vi "DSC TSV to PGSQL Choose Column Dialog.vi"(8 "error in":errorcluster, 9 "Message":string, 10 "DSC":string, 11 "Item Names":string[](array[string])) -> (0 "error out":errorcluster, 3 "Selection":string)   [LabVIEW 2019]
uses:
  <vilib>/ErrorRing/Error Ring.xnode
panel:
  in  "CANCEL":bool
  in  "Listbox":i32(listbox)
  in  "OK":bool
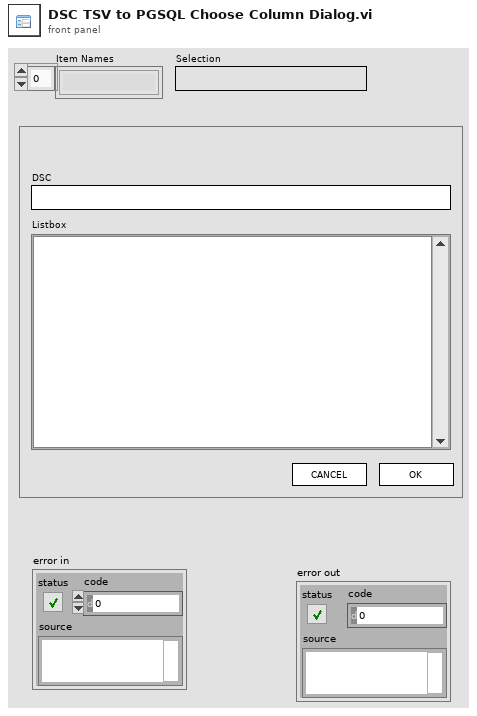
[diagram p1: front panel]
types:
  T1 = enum32{"Invalid", "Standard", "Closed", "Hidden", "Minimized", "Maximized"}
  T2 = enum32{"invalid app kind", "Development System", "Run Time System", "Student Edition", "Embedded LabVIEW", "Evaluation", "Custom"}
  T3 = cluster{"Core":cluster{"Current VI Reference":refnum<vi>, "Close Panel on Exit?":bool}, "Cancel?":bool, "Your string data":string}
  T4 = cluster{"Current VI Reference":refnum<vi>, "Close Panel on Exit?":bool}
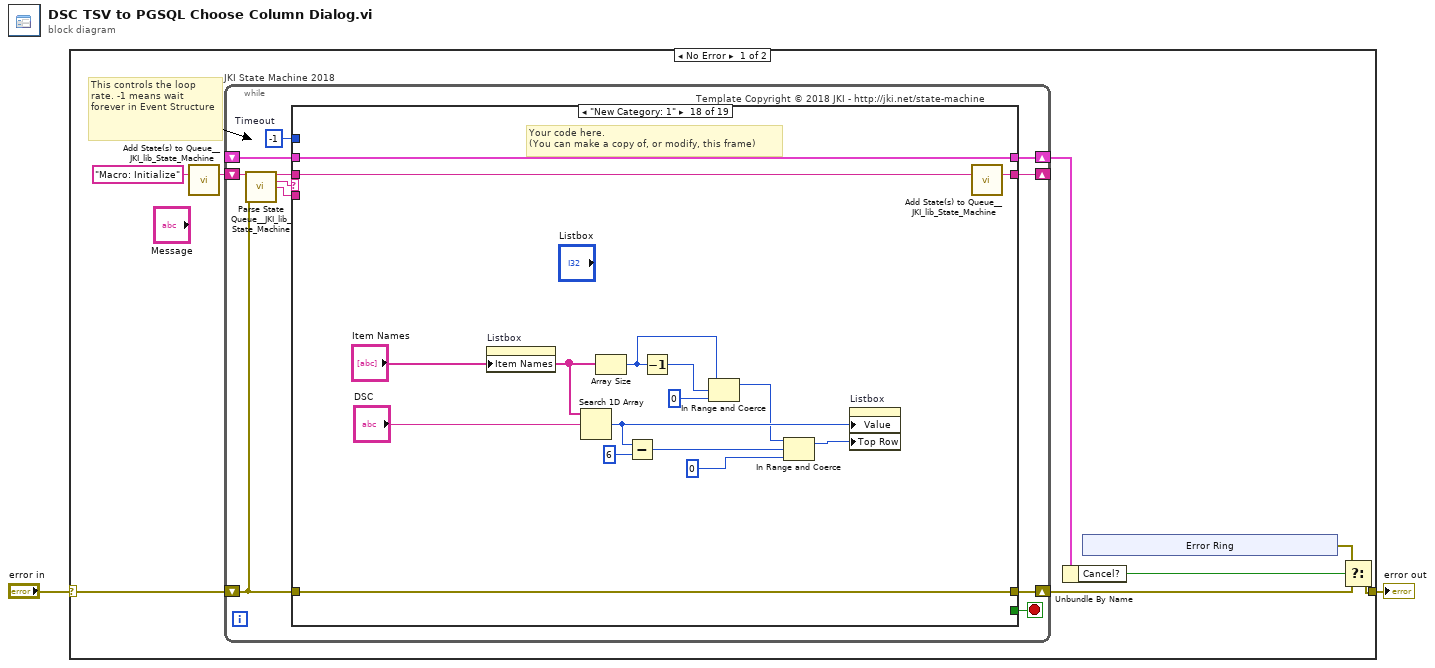
[diagram p0: block diagram]
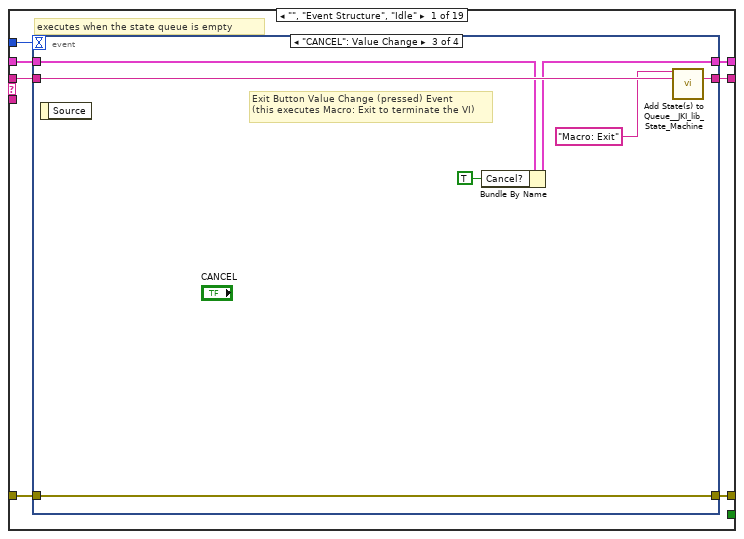
[diagram p2: hidden frame]
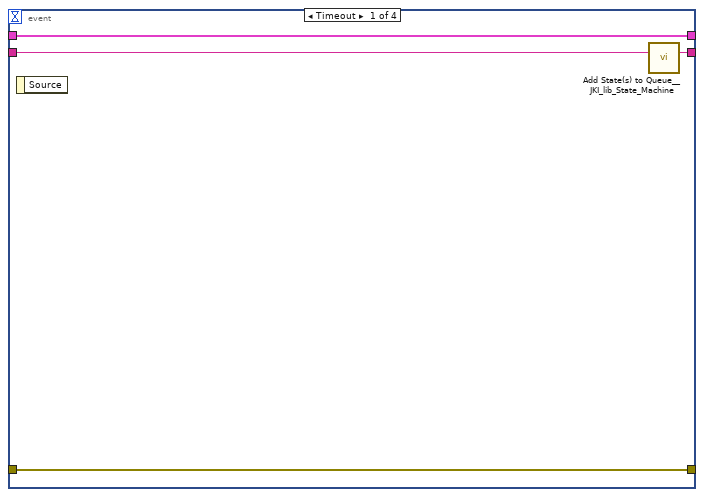
[diagram p3: hidden frame]
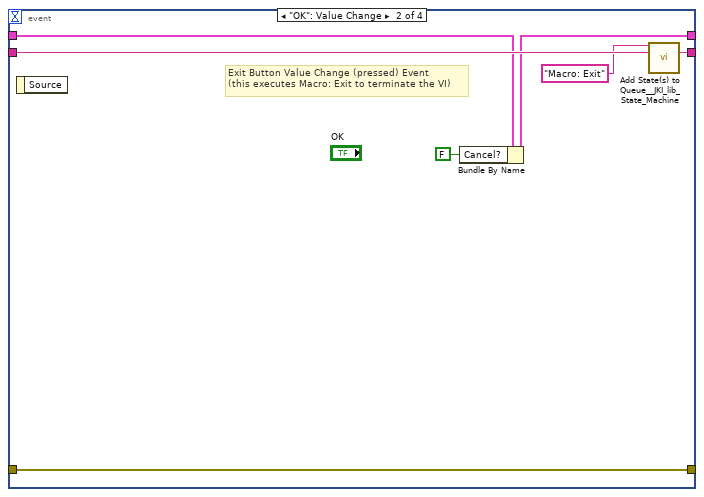
[diagram p4: hidden frame]
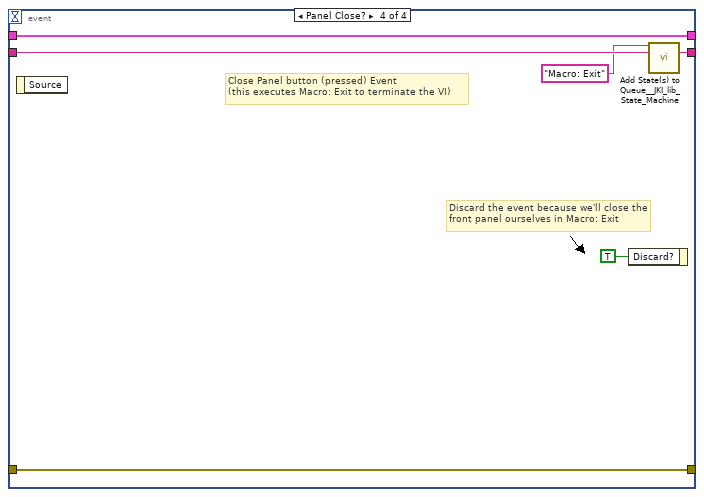
[diagram p5: hidden frame]
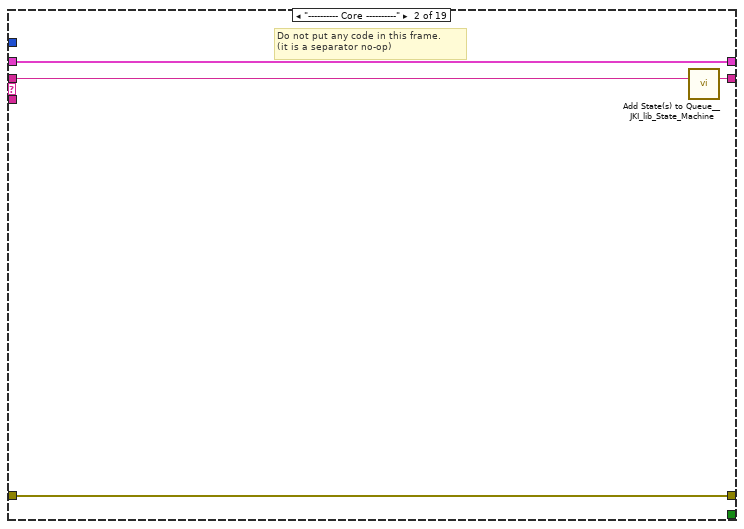
[diagram p6: hidden frame]
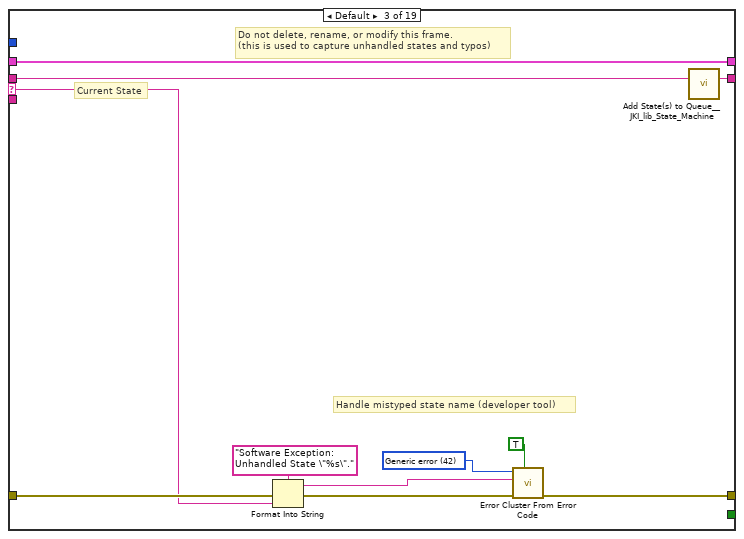
[diagram p7: hidden frame]
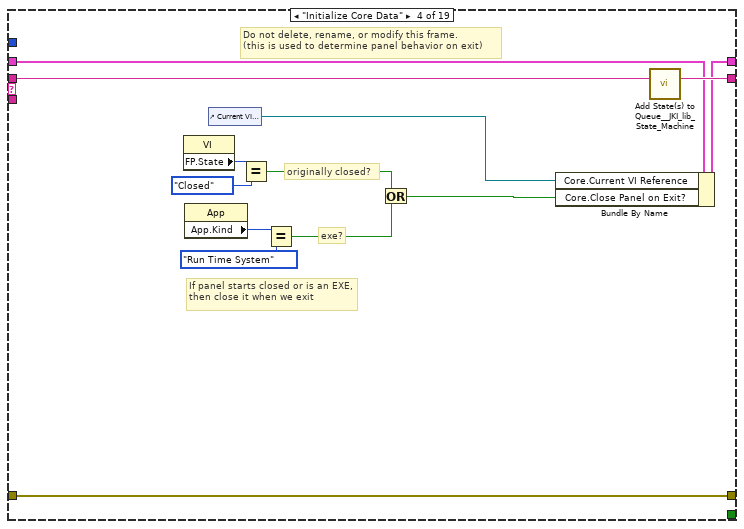
[diagram p8: hidden frame]
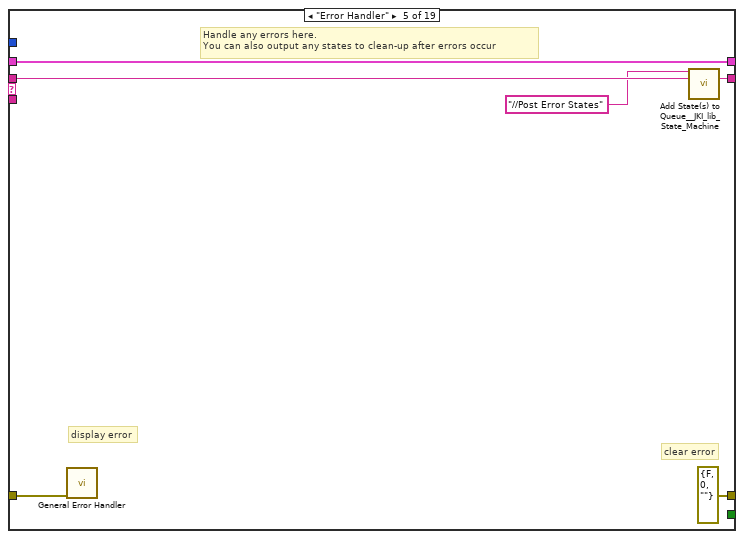
[diagram p9: hidden frame]
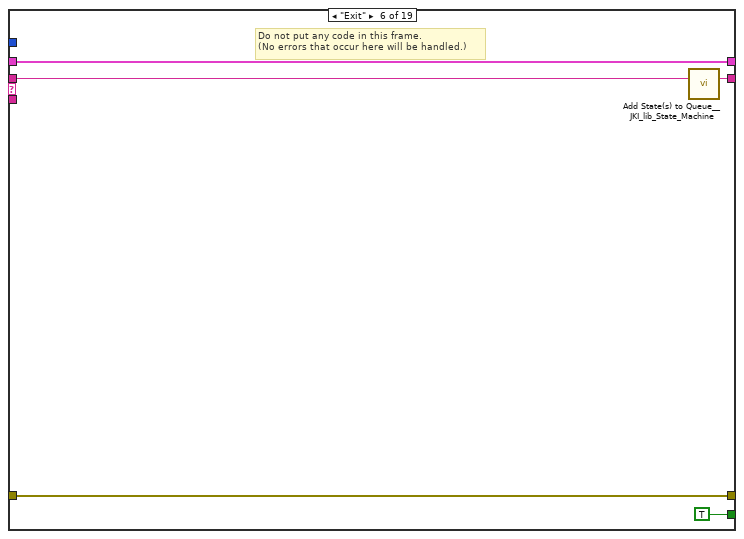
[diagram p10: hidden frame]
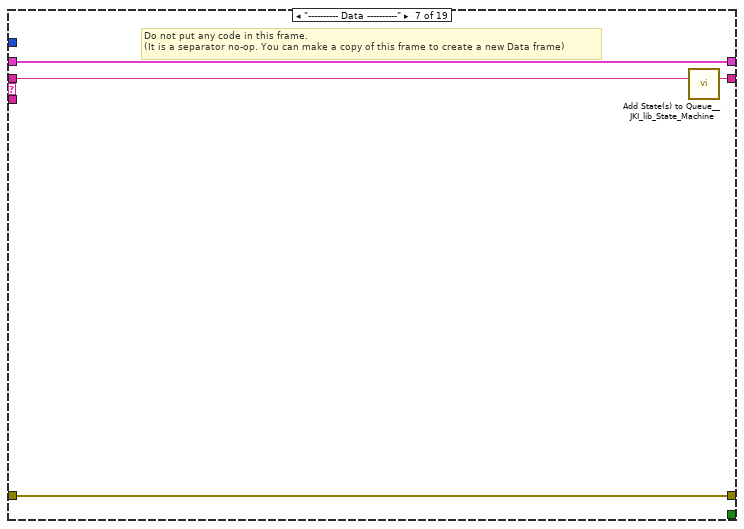
[diagram p11: hidden frame]
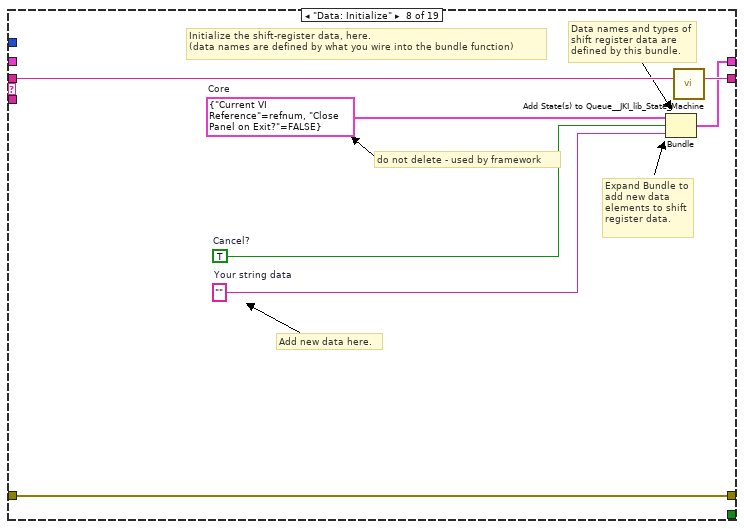
[diagram p12: hidden frame]
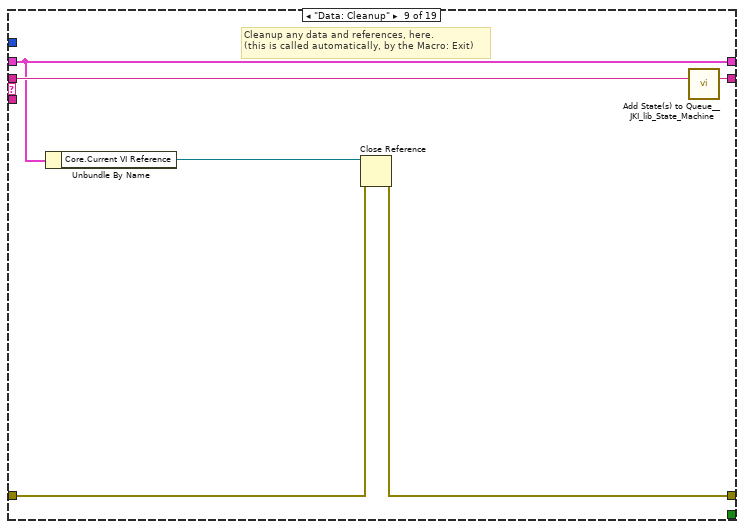
[diagram p13: hidden frame]
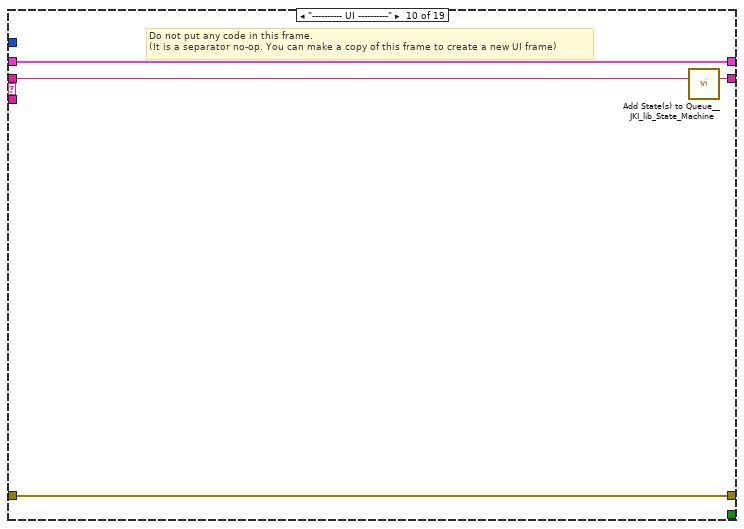
[diagram p14: hidden frame]
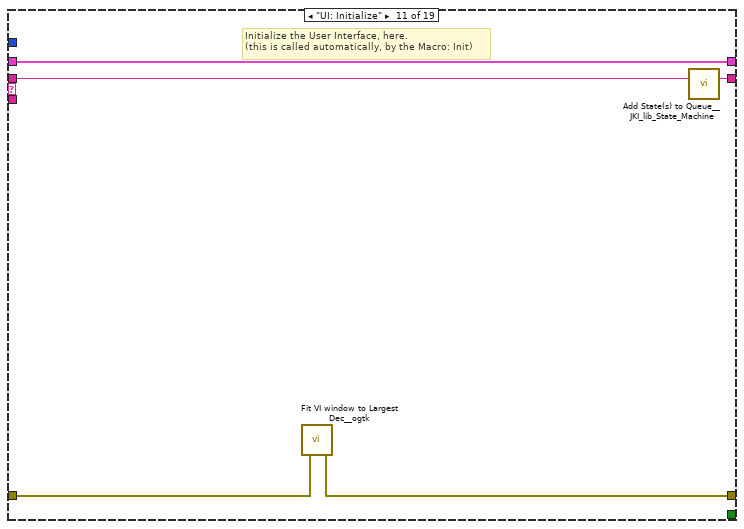
[diagram p15: hidden frame]
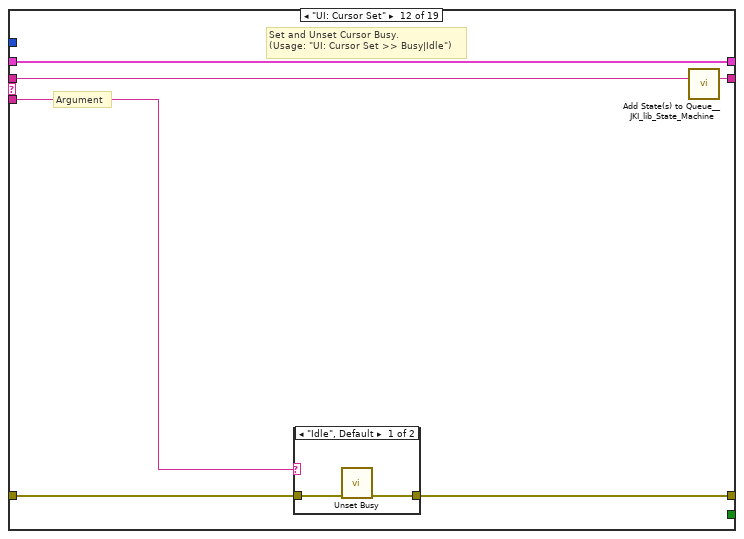
[diagram p16: hidden frame]
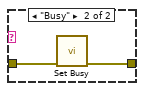
[diagram p17: hidden frame]
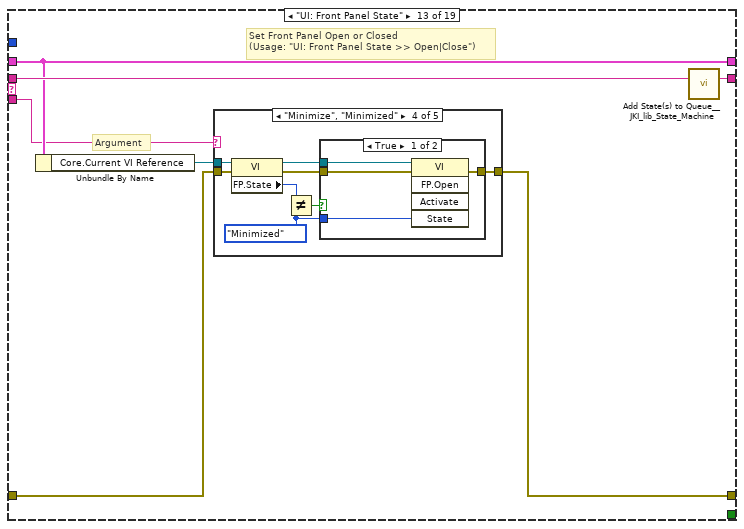
[diagram p18: hidden frame]
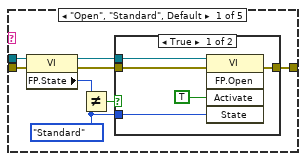
[diagram p19: hidden frame]
diagram:
  n1 = case shown="No Error" "error in" {
    selector: "error in" -> [w3 w250]
    tunnel: [w5 w250] -> w2
    frame No Error {
      # "This controls the loop rate. -1 means wait forever in Event Structure"
      n2 = call <vilib>:"Add State(s) to Queue__JKI_lib_State_Machine.vi"("State(s) in (\"\")"="Macro: Initialize") -> ("States Out"=w10:string)  [unwired: 14 in]
      n3 = while "JKI State Machine 2018" {
        shift-right: [w18] -> w8
        shift-left: _ -> [w17]
        shift-right: [w21] -> w6
        shift-left: w3 -> [w15]
        shift-right: [w20] -> _
        shift-left: w10 -> [w22]
        stop <- w19 stop-if-true
        w16 = -1  # Timeout
        # "Template Copyright © 2018 JKI - http://jki.net/state-machine"
        n4 = call <vilib>:"Parse State Queue__JKI_lib_State_Machine.vi"("State Queue"=w22, "Error In (no error)"=w15) -> ("Remaining States"=w24:string, "Current State"=w25:string, "Arguments"=w23:string)  [unwired: 11 in]
        n5 = case shown="\"New Category: 1\"" w25 {
          selector: w25 -> [_ _ w61 _ _ _ _ _ _ _ _ _ _ _ _ _ _ _ _]
          tunnel: w24 -> [w32 w60 w65 w84 w90 w95 w99 w106 w112 w116 w121 w127 w138 w207 w212 w223 w227 w242 w249]
          tunnel: w23 -> [_ _ _ _ _ _ _ _ _ _ _ w122 w132 _ _ _ _ _ _]
          tunnel: w17 -> [w30 w57 w63 w77 w88 w93 w96 _ w107 w113 w119 w125 w134 w204 w209 w220 w224 w239 w246]
          tunnel: [w29 w58 w67 w81 errorcluster {"status"=FALSE, "code"=0, "source"=""} ("error in") w92 w97 w103 w108 w114 w118 w123 w135 w205 w210 w221 w225 w240 w247] -> w21
          tunnel: w15 -> [w28 w58 w66 w81 w85 w92 w97 w103 w109 w114 w117 w124 w136 w205 w210 w221 w225 w240 w247]
          tunnel: [w31 w59 w64 w83 w89 w94 w98 w105 w111 w115 w120 w126 w137 w206 w211 w222 w226 w241 w248] -> w20
          tunnel: [_ _ _ _ _ TRUE _ _ _ _ _ _ _ _ _ _ _ _ _] -> w19
          tunnel: [w27 w57 w63 w82 w88 w93 w96 w104 w107 w113 w119 w125 w134 w204 w209 w220 w224 w239 w246] -> w18
          tunnel: w16 -> [w26 _ _ _ _ _ _ _ _ _ _ _ _ _ _ _ _ _ _]
          frame "", "Event Structure", "Idle" {
            # "executes when the state queue is empty"
            n6 = event shown="[2] \"CANCEL\": Value Change" {
              selector: _ -> [_ _ _ _]
              dyn-events: _ -> [_ _ _ _]
              timeout: w26 -> [_ _ _ _]
              tunnel: w32 -> [w36 w43 w50 w56]
              tunnel: [w35 w42 w49 w55] -> w31
              tunnel: w30 -> [w33 w37 w44 w53]
              tunnel: [w34 w41 w48 w54] -> w29
              tunnel: w28 -> [w34 w41 w48 w54]
              tunnel: [w33 w38 w45 w53] -> w27
              event Timeout {
                n7 = event-data() -> ()  [unwired: 1 in, 1 out]
                n8 = call <vilib>:"Add State(s) to Queue__JKI_lib_State_Machine.vi"("State(s) in (\"\")"=w36) -> ("States Out"=w35:string)  [unwired: 14 in]
              }
              event "OK": Value Change {
                # "Exit Button Value Change (pressed) Event\n(this executes Macro: Exit to terminate the VI)"
                n9 = event-data() -> ()  [unwired: 1 in, 1 out]
                n10 = Bundle By Name(cluster=w37, "Cancel?"=FALSE) -> (w38:T3)
                n11 = call <vilib>:"Add State(s) to Queue__JKI_lib_State_Machine.vi"("State(s) in Front (\"\")"="Macro: Exit", "State(s) in (\"\")"=w43) -> ("States Out"=w42:string)  [unwired: 13 in]
              }
              event "CANCEL": Value Change {
                # "Exit Button Value Change (pressed) Event\n(this executes Macro: Exit to terminate the VI)"
                n12 = event-data() -> ()  [unwired: 1 in, 1 out]
                n13 = Bundle By Name(cluster=w44, "Cancel?"=TRUE) -> (w45:T3)
                n14 = call <vilib>:"Add State(s) to Queue__JKI_lib_State_Machine.vi"("State(s) in Front (\"\")"="Macro: Exit", "State(s) in (\"\")"=w50) -> ("States Out"=w49:string)  [unwired: 13 in]
              }
              event Panel Close? {
                # "Discard the event because we'll close the front panel ourselves in Macro: Exit"
                # "Close Panel button (pressed) Event\n(this executes Macro: Exit to terminate the VI)"
                n15 = event-data() -> ()  [unwired: 1 in, 1 out]
                n16 = event-data("Discard?"=TRUE) -> ()  [unwired: 1 in, 1 out]
                n17 = call <vilib>:"Add State(s) to Queue__JKI_lib_State_Machine.vi"("State(s) in Front (\"\")"="Macro: Exit", "State(s) in (\"\")"=w56) -> ("States Out"=w55:string)  [unwired: 13 in]
              }
            }
          }
          frame "---------- Core ----------" {
            # "Do not put any code in this frame.\n(it is a separator no-op)"
            n18 = call <vilib>:"Add State(s) to Queue__JKI_lib_State_Machine.vi"("State(s) in (\"\")"=w60) -> ("States Out"=w59:string)  [unwired: 14 in]
          }
          frame Default {
            w70 = 42 items=["No error", "Argument error", "Memory is full", "Out of zone", "End of file", "File already open", "Generic file I/O error", "File not found", "File permission error", "Disk is full", "Duplicate path", "Too many files open", "System feature not enabled", "Resource file not found", "Cannot add resource", "Resource not found", "Image not found", "Image memory error", "Pen does not exist", "Config type invalid", "Config token not found", "Config parse error", "Config memory error", "Bad external code format", "Bad external code offset", "External code not present", "Null window", "Destroy window error", "Null menu", "Print aborted", "Bad print record", "Print driver error", "Windows error during printing", "Memory error during printing", "Print dialog error", "Generic print error", "Invalid device refnum", "Device not found", "Device parameter error", "Device unit error", "Cannot open device", "Device call aborted", "Generic error", "Cancelled by user", "Object ID too low", "Object ID too high", "Object not in heap", "Unknown heap", "Unknown object (invalid DefProc)", "Unknown object (DefProc not in table)", "Message out of range", "Invalid (null) method", "Unknown message", "Manager call not supported", "Bad address", "Network operation in progress", "Network operation timed out", "Connection is busy", "Network attribute not supported", "Network error", "Address in use", "System out of memory", "Connection aborted", "Connection refused", "Not connected", "Already connected", "Connection closed", "Initialization error (interapplication manager)", "Bad occurrence", "Wait on unbound occurrence handler", "Occurrence queue overflow", "Datalog type conflict", "Unused", "Unrecognized type (interapplication manager)", "Memory corrupt", "Failed to make temporary DLL", "Old CIN version", "Drag socket not found", "Failed to load drop-object", "Failed to register OLE object", "Failed to release OLE object", "Format specifier type mismatch", "Unknown format specifier", "Too few format specifiers", "Too many format specifiers", "Scan failed", "Newer CIN version", "Error converting to variant", "Runtime menu error", "Password tampered", "Variant attribute not found", "Incompatible variant data type", "Event data is not available", "Event Store is not present", "Occurrence is not found", "Event Queue is not created", "Event info is not available", "Refnum passed is NULL", "Error retrieving Class GUID", "Error retrieving CoClass GUID", "Error retrieving TypeLib GUID.", "Bad built application magic bytes.", "Specific driver is different from the specific driver associated with the Logical Name.", "There is no session opened to the class driver.", "Max Error", "MAX - Error with config objects", "MAX - Error loading configuration", "MAX - Group not supported"]
            # "Current State"
            # "Do not delete, rename, or modify this frame.\n(this is used to capture unhandled states and typos)"
            # "Handle mistyped state name (developer tool)"
            n19 = Format Into String(format string="Software Exception: Unhandled State \"%s\"." ("message"), error in=w66, w61) -> (resulting string=w69:string, error out=w68:errorcluster)  [unwired: 1 in]
            n20 = call <vilib>:"Error Cluster From Error Code.vi"("show call chain? (False)"=TRUE, "error in (no error)"=w68, "error message (\"\")"=w69, "error code (0)"=w70) -> ("error out"=w67:errorcluster)  [unwired: 5 in]
            n21 = call <vilib>:"Add State(s) to Queue__JKI_lib_State_Machine.vi"("State(s) in (\"\")"=w65) -> ("States Out"=w64:string)  [unwired: 14 in]
          }
          frame "Initialize Core Data" {
            # "Do not delete, rename, or modify this frame.\n(this is used to determine panel behavior on exit)"
            # "originally closed?"
            # "exe?"
            # "If panel starts closed or is an EXE, then close it when we exit"
            n22 = property class="VI"() -> ("FP.State"=w74:T1)  [unwired: 2 in, 2 out]
            n23 = property class="App"() -> ("App.Kind"=w80:T2)  [unwired: 2 in, 2 out]
            n24 = control-ref of="Current VI Reference"() -> (w75:refnum<vi>)
            n25 = Equal?(x=w74, y=T1."Closed" ("Front Panel Window:State")) -> (x = y?=w72:bool)
            n26 = Equal?(x=w80, y=T2."Run Time System" ("Application:Kind")) -> (x = y?=w78:bool)
            n27 = Or(x=w72, y=w78) -> (x .or. y?=w76:bool)
            n28 = Bundle By Name(cluster=w77, "Core.Current VI Reference"=w75, "Core.Close Panel on Exit?"=w76) -> (w82:T3)
            n29 = call <vilib>:"Add State(s) to Queue__JKI_lib_State_Machine.vi"("State(s) in (\"\")"=w84) -> ("States Out"=w83:string)  [unwired: 14 in]
          }
          frame "Error Handler" {
            # "display error"
            # "clear error"
            # "Handle any errors here.\nYou can also output any states to clean-up after errors occur"
            n30 = call <vilib>:"General Error Handler.vi"("error in (no error)"=w85) -> ()  [unwired: 10 in, 5 out]
            n31 = call <vilib>:"Add State(s) to Queue__JKI_lib_State_Machine.vi"("State(s) in Front (\"\")"="//Post Error States", "State(s) in (\"\")"=w90) -> ("States Out"=w89:string)  [unwired: 13 in]
          }
          frame "Exit" {
            # "Do not put any code in this frame.\n(No errors that occur here will be handled.)"
            n32 = call <vilib>:"Add State(s) to Queue__JKI_lib_State_Machine.vi"("State(s) in (\"\")"=w95) -> ("States Out"=w94:string)  [unwired: 14 in]
          }
          frame "---------- Data ----------" {
            # "Do not put any code in this frame.\n(It is a separator no-op. You can make a copy of this frame to create a new Data frame)"
            n33 = call <vilib>:"Add State(s) to Queue__JKI_lib_State_Machine.vi"("State(s) in (\"\")"=w99) -> ("States Out"=w98:string)  [unwired: 14 in]
          }
          frame "Data: Initialize" {
            w100 = T4 {"Current VI Reference"=refnum, "Close Panel on Exit?"=FALSE}  # Core
            w102 = TRUE  # Cancel?
            w101 = ""  # Your string data
            # "do not delete - used by framework"
            # "Expand Bundle to add new data elements to shift register data."
            # "Add new data here."
            # "Data names and types of shift register data are defined by this bundle."
            # "Initialize the shift-register data, here.\n(data names are defined by what you wire into the bundle function)"
            n34 = Bundle("Core"=w100, "Cancel?"=w102, "Your string data"=w101) -> (w104:T3)  [unwired: 1 in]
            n35 = call <vilib>:"Add State(s) to Queue__JKI_lib_State_Machine.vi"("State(s) in (\"\")"=w106) -> ("States Out"=w105:string)  [unwired: 14 in]
          }
          frame "Data: Cleanup" {
            # "Cleanup any data and references, here.\n(this is called automatically, by the Macro: Exit)"
            n36 = Unbundle By Name(w107) -> ("Core.Current VI Reference"=w110:refnum<vi>)
            n37 = Close Reference(reference=w110, error in (no error)=w109) -> (error out=w108:errorcluster)
            n38 = call <vilib>:"Add State(s) to Queue__JKI_lib_State_Machine.vi"("State(s) in (\"\")"=w112) -> ("States Out"=w111:string)  [unwired: 14 in]
          }
          frame "---------- UI ----------" {
            # "Do not put any code in this frame.\n(It is a separator no-op. You can make a copy of this frame to create a new UI frame)"
            n39 = call <vilib>:"Add State(s) to Queue__JKI_lib_State_Machine.vi"("State(s) in (\"\")"=w116) -> ("States Out"=w115:string)  [unwired: 14 in]
          }
          frame "UI: Initialize" {
            # "Initialize the User Interface, here.\n(this is called automatically, by the Macro: Init)"
            n40 = call <userlib>:"Fit VI window to Largest Dec__ogtk.vi"("error in (no error)"=w117) -> ("error out"=w118:errorcluster)  [unwired: 5 in, 1 out]
            n41 = call <vilib>:"Add State(s) to Queue__JKI_lib_State_Machine.vi"("State(s) in (\"\")"=w121) -> ("States Out"=w120:string)  [unwired: 14 in]
          }
          frame "UI: Cursor Set" {
            # "Argument"
            # "Set and Unset Cursor Busy.\n(Usage: \"UI: Cursor Set >> Busy|Idle\")"
            n42 = case shown="\"Idle\", Default" w122 {
              tunnel: w124 -> [w129 w131]
              tunnel: [w128 w130] -> w123
              frame "Idle", Default {
                n43 = call <vilib>:"Unset Busy.vi"("error in (no error)"=w129) -> ("error out"=w128:errorcluster)  [unwired: 10 in]
              }
              frame "Busy" {
                n44 = call <vilib>:"Set Busy.vi"("error in (no error)"=w131) -> ("error out"=w130:errorcluster)  [unwired: 9 in, 1 out]
              }
            }
            n45 = call <vilib>:"Add State(s) to Queue__JKI_lib_State_Machine.vi"("State(s) in (\"\")"=w127) -> ("States Out"=w126:string)  [unwired: 14 in]
          }
          frame "UI: Front Panel State" {
            # "Argument"
            # "Set Front Panel Open or Closed\n(Usage: \"UI: Front Panel State >> Open|Close\")"
            n46 = Unbundle By Name(w134) -> ("Core.Current VI Reference"=w133:refnum<vi>)
            n47 = case shown="\"Minimize\", \"Minimized\"" w132 {
              tunnel: w136 -> [w144 w159 w170 w183 w196]
              tunnel: [w146 w160 w172 w185 w198] -> w135
              tunnel: w133 -> [w145 w157 w171 w184 w197]
              frame "Open", "Standard", Default {
                w139 = T1."Standard" ("State")
                n48 = property class="VI"(reference=w145, error in=w144) -> (reference out=w142:refnum<vi>, error out=w143:errorcluster, "FP.State"=w141:T1)
                n49 = Not Equal?(x=w141, y=w139) -> (x != y?=w140:bool)
                n50 = case shown="True" w140 {
                  tunnel: [w150 w152] -> w146
                  tunnel: w143 -> [w149 w152]
                  tunnel: w142 -> [w148 _]
                  tunnel: w139 -> [w147 _]
                  frame True {
                    n51 = invoke class="VI" method="FP.Open"(reference=w148, error in=w149, "Activate"=TRUE, "State"=w147) -> (error out=w150:errorcluster)  [unwired: 1 in, 4 out]
                  }
                  frame False {
                  }
                }
              }
              frame "Close", "Closed" {
                n52 = property class="VI"(reference=w157, error in=w159) -> (reference out=w156:refnum<vi>, error out=w158:errorcluster, "FP.State"=w154:T1)
                n53 = Not Equal?(x=w154, y=T1."Closed" ("Front Panel Window:State")) -> (x != y?=w153:bool)
                n54 = case shown="True" w153 {
                  tunnel: [w161 w164] -> w160
                  tunnel: w158 -> [w161 w163]
                  tunnel: w156 -> [_ w162]
                  frame False {
                  }
                  frame True {
                    n55 = invoke class="VI" method="FP.Close"(reference=w162, error in=w163) -> (error out=w164:errorcluster)  [unwired: 1 in, 2 out]
                  }
                }
              }
              frame "Hidden", "Hide" {
                w165 = T1."Hidden" ("State")
                n56 = property class="VI"(reference=w171, error in=w170) -> (reference out=w168:refnum<vi>, error out=w169:errorcluster, "FP.State"=w167:T1)
                n57 = Not Equal?(x=w167, y=w165) -> (x != y?=w166:bool)
                n58 = case shown="True" w166 {
                  tunnel: [w176 w177] -> w172
                  tunnel: w169 -> [w175 w177]
                  tunnel: w168 -> [w174 _]
                  tunnel: w165 -> [w173 _]
                  frame True {
                    n59 = invoke class="VI" method="FP.Open"(reference=w174, error in=w175, "State"=w173) -> (error out=w176:errorcluster)  [unwired: 2 in, 4 out]
                  }
                  frame False {
                  }
                }
              }
              frame "Minimize", "Minimized" {
                w178 = T1."Minimized" ("State")
                n60 = property class="VI"(reference=w184, error in=w183) -> (reference out=w181:refnum<vi>, error out=w182:errorcluster, "FP.State"=w180:T1)
                n61 = Not Equal?(x=w180, y=w178) -> (x != y?=w179:bool)
                n62 = case shown="True" w179 {
                  tunnel: [w189 w190] -> w185
                  tunnel: w182 -> [w188 w190]
                  tunnel: w181 -> [w187 _]
                  tunnel: w178 -> [w186 _]
                  frame True {
                    n63 = invoke class="VI" method="FP.Open"(reference=w187, error in=w188, "State"=w186) -> (error out=w189:errorcluster)  [unwired: 2 in, 4 out]
                  }
                  frame False {
                  }
                }
              }
              frame "Maximize", "Maximized" {
                w191 = T1."Maximized" ("State")
                n64 = property class="VI"(reference=w197, error in=w196) -> (reference out=w194:refnum<vi>, error out=w195:errorcluster, "FP.State"=w193:T1)
                n65 = Not Equal?(x=w193, y=w191) -> (x != y?=w192:bool)
                n66 = case shown="True" w192 {
                  tunnel: [w202 w203] -> w198
                  tunnel: w195 -> [w201 w203]
                  tunnel: w194 -> [w200 _]
                  tunnel: w191 -> [w199 _]
                  frame True {
                    n67 = invoke class="VI" method="FP.Open"(reference=w200, error in=w201, "State"=w199) -> (error out=w202:errorcluster)  [unwired: 2 in, 4 out]
                  }
                  frame False {
                  }
                }
              }
            }
            n68 = call <vilib>:"Add State(s) to Queue__JKI_lib_State_Machine.vi"("State(s) in (\"\")"=w138) -> ("States Out"=w137:string)  [unwired: 14 in]
          }
          frame "---------- Macro ----------" {
            # "Do not put any code in this frame.\n(It is a separator no-op. You can make a copy of this frame to create a new Macro frame)"
            n69 = call <vilib>:"Add State(s) to Queue__JKI_lib_State_Machine.vi"("State(s) in (\"\")"=w207) -> ("States Out"=w206:string)  [unwired: 14 in]
          }
          frame "Macro: Initialize" {
            w208 = "Data: Initialize\nInitialize Core Data\nUI: Initialize\nUI: Front Panel State >> Open\nNew Category: 1"  # Data: Initialize Initialize Core Data UI: Initialize UI: Front Panel State >> Open New Category: 1
            # "Initialization Macro\n(This is called once, when the VI starts)"
            n70 = call <vilib>:"Add State(s) to Queue__JKI_lib_State_Machine.vi"("State(s) in Front (\"\")"=w208, "State(s) in (\"\")"=w212) -> ("States Out"=w211:string)  [unwired: 13 in]
          }
          frame "Macro: Exit" {
            # "Exit Macro\n(This is called once, when the VI exits)"
            n71 = Unbundle By Name(w220) -> ("Core.Close Panel on Exit?"=w219:bool)
            n72 = Select(t="UI: Front Panel State >> Close", s=w219, f="") -> (s? t:f=w216:string)
            n73 = call <vilib>:"Add State(s) to Queue__JKI_lib_State_Machine.vi"("State(s) in Front (\"\")"="New Category: 2" ("State(s) in Front (\"\")"), "State(s) in (\"\")"=w216, "State(s) at Back (\"\")"="Data: Cleanup\nExit") -> ("States Out"=w214:string)  [unwired: 12 in]
            n74 = call <vilib>:"Add State(s) to Queue__JKI_lib_State_Machine.vi"("State(s) in Front (\"\")"=w214, "State(s) in (\"\")"=w223) -> ("States Out"=w222:string)  [unwired: 13 in]
          }
          frame "---------- New Category ----------" {
            # "Template Separator\n(You can make a copy of, or modify, this frame)"
            n75 = call <vilib>:"Add State(s) to Queue__JKI_lib_State_Machine.vi"("State(s) in (\"\")"=w227) -> ("States Out"=w226:string)  [unwired: 14 in]
          }
          frame "New Category: 1" {
            # "Your code here.\n(You can make a copy of, or modify, this frame)"
            n76 = property on="Listbox" class="LstBox (strict)"("Item Names"="Item Names") -> ()  [unwired: 2 in, 2 out]
            n77 = Search 1D Array(1D array="Item Names", element="DSC") -> (index of element=w235:i32)  [unwired: 1 in]
            n78 = Array Size(array="Item Names") -> (size(s)=w230:i32)
            n79 = Subtract(x=w235, y=6) -> (x-y=w232:i32)
            n80 = Decrement(x=w230) -> (x-1=w229:i32)
            n81 = In Range and Coerce(upper limit=w230, x=w229, lower limit=0) -> (coerced(x)=w228:i32)  [unwired: 1 out]
            n82 = In Range and Coerce(upper limit=w228, x=w232, lower limit=0) -> (coerced(x)=w233:i32)  [unwired: 1 out]
            n83 = property on="Listbox" class="LstBox (strict)"("Value"=w235, "Top Row"=w233) -> ()  [unwired: 2 in, 2 out]
            n84 = call <vilib>:"Add State(s) to Queue__JKI_lib_State_Machine.vi"("State(s) in (\"\")"=w242) -> ("States Out"=w241:string)  [unwired: 14 in]
          }
          frame "New Category: 2" {
            # "Your code here.\n(You can make a copy of, or modify, this frame)"
            n85 = property on="Listbox" class="LstBox (strict)"() -> ("Item Names"=w245:string[], "Value"=w244:i32)  [unwired: 2 in, 2 out]
            n86 = Index Array(array=w245, index=w244) -> (element=→"Selection":string)
            n87 = call <vilib>:"Add State(s) to Queue__JKI_lib_State_Machine.vi"("State(s) in (\"\")"=w249) -> ("States Out"=w248:string)  [unwired: 14 in]
          }
        }
      }
      n88 = Unbundle By Name(w8) -> ("Cancel?"=w7:bool)
      n89 = xnode "Error Ring"() -> ("error out"=w4:errorcluster)
      n90 = Select(t=w4, s=w7, f=w6) -> (s? t:f=w5:errorcluster)
    }
    frame Error {
    }
  }
  "error out" <- w2
